vi "test_ParseSolutionFile_AddPackedLibs.vi"() -> (3 "Pass?":bool)   [LabVIEW 2019, in "Tests.SolutionBuilder.lvlib"]
uses:
  Tests.SolutionBuilder.lvlib
  SolutionBuilder/SolutionBuilder.lvclass
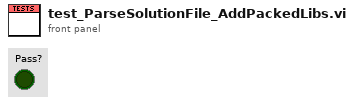
[diagram p1: front panel]
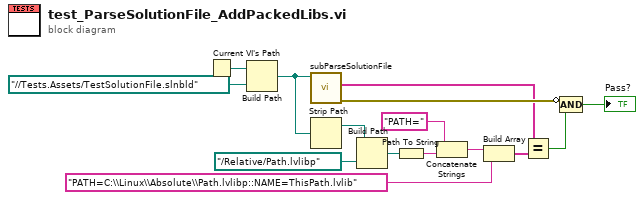
[diagram p0: block diagram]
diagram:
  n1 = Current VI's Path() -> (path=w14:path)
  n2 = Build Path(base path=w14, name or relative path=path "../../Tests.Assets/TestSolutionFile.slnbld" ("Path")) -> (appended path=w10:path)
  n3 = call "subParseSolutionFile.vi"("Solution file"=w10) -> ("error out"=w9:errorcluster, "Lib definition strings"=w7:string[])  [unwired: 7 in, 2 out]
  n4 = Strip Path(path=w10) -> (stripped path=w11:path)  [unwired: 1 out]
  n5 = Build Path(base path=w11, name or relative path=path "../Relative/Path.lvlibp" ("Path")) -> (appended path=w4:path)
  n6 = Path To String(path=w4) -> (string=w3:string)
  n7 = Concatenate Strings("PATH=" ("string"), w3) -> (w1:string)
  n8 = Build Array(w1, "PATH=C:\\Linux\\Absolute\\Path.lvlibp::NAME=ThisPath.lvlib") -> (w5:string[])
  n9 = Equal?(x=w7, y=w5) -> (x = y?=w8:bool)
  n10 = Compound Arithmetic op=AND(invert w9, w8) -> (→"Pass?":bool)
